vi "VDP.vi"(5 "Settling time":u32=2, 6 "Enable Output (T: Enable)":bool, 8 "error in (no error)":errorcluster, 9 "VISA scanner":refnum<visa-resource-name>="GPIB0::10::INSTR", 10 "VISA nanoVM":refnum<visa-resource-name>="GPIB0::12::INSTR", 11 "VISA current":refnum<visa-resource-name>="K2401") -> (0 "error out":errorcluster, 1 "sheet resistance":dbl)   [LabVIEW 2019]
panel:
  out "Array":sgl[](array[numeric])
  out "VISA scanner out":refnum<visa-resource-name>
  out "VISA nanovoltmeter out":refnum<visa-resource-name>
  out "VISA current out":refnum<visa-resource-name>
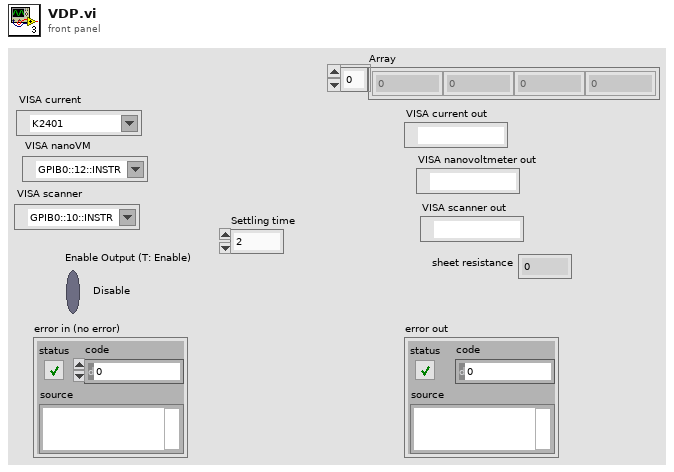
[diagram p1: front panel]
types:
  T1 = cluster{"error":bool, "code":i32, "source":string}
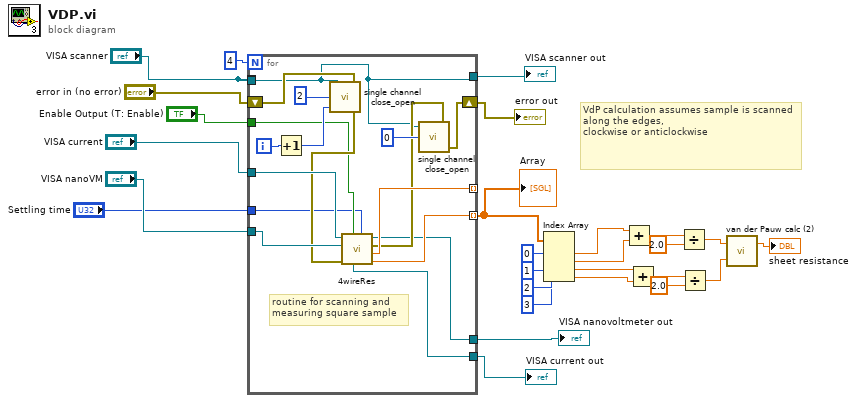
[diagram p0: block diagram]
diagram:
  # "VdP calculation assumes sample is scanned along the edges, \nclockwise or anticlockwise"
  n1 = for {
    N: 4 -> [_]
    tunnel: "VISA current" -> [w44]
    tunnel: "VISA nanoVM" -> [w43]
    tunnel: "VISA scanner" -> [_]
    tunnel: "VISA scanner" -> [w31]
    tunnel: "Enable Output (T: Enable)" -> [w39]
    tunnel: [w38] -> _ mode=indexing
    tunnel: [w37] -> w5 mode=indexing
    shift-right: [w32] -> w22
    shift-left: "error in (no error)" -> [w36]
    tunnel: [w31] -> w4
    tunnel: [w30] -> w3
    tunnel: [w29] -> w2
    tunnel: "Settling time" -> [w28]
    i -> [w35]
    # "routine for scanning and \nmeasuring square sample"
    n2 = Increment(x=w35) -> (x+1=w41:i32)
    n3 = call "single channel close_open.vi"("error in"=w36, "channel"=w41, "open all 0 / close 2"=i16 2, "VISA resource name"=w31) -> ("error out"=w40:T1)  [unwired: 1 in]
    n4 = call "4wireRes.vi"("Settling time"=w28, "Enable Output (T: Enable)"=w39, "error in (no error)"=w40, "VISA nanoVM"=w43, "VISA current"=w44) -> ("R4pt"=w37:dbl, "R2pt"=w38:sgl, "error out"=w33:errorcluster, "VISA nanovoltmeter out"=w30:refnum<visa-resource-name>, "VISA current out"=w29:refnum<visa-resource-name>)  [unwired: 2 in]
    n5 = call "single channel close_open.vi"("error in"=w33, "open all 0 / close 2"=i16 0, "VISA resource name"=w31) -> ("error out"=w32:T1)  [unwired: 2 in]
  }
  "VISA current out" <- w2
  "error out" <- w22
  "VISA nanovoltmeter out" <- w3
  "VISA scanner out" <- w4
  "Array" <- w5
  n6 = Index Array(array=w5, index #1=0 ("index"), index #2=1 ("index"), index #3=2 ("index"), index #4=3 ("index")) -> (element #1=w16:dbl, element #2=w9:dbl, element #3=w10:dbl, element #4=w15:dbl)
  n7 = Add(x=w16, y=w9) -> (x+y=w14:dbl)
  n8 = Add(x=w10, y=w15) -> (x+y=w13:dbl)
  n9 = Divide(x=w14, y=2.0) -> (x/y=w8:dbl)
  n10 = Divide(x=w13, y=2.0) -> (x/y=w7:dbl)
  n11 = call "van der Pauw calc (2).vi"("horizontal resistance"=w7, "vertical resistance"=w8) -> ("Sheet resistance"=→"sheet resistance":dbl)  [unwired: 1 in]
